vi "GitLog-to-CommitCluster.vi"(3 "Git Log In":string) -> (1 "Array":T1[](array[typedef]))   [LabVIEW 2013]
uses:
  CommitCluster.ctl
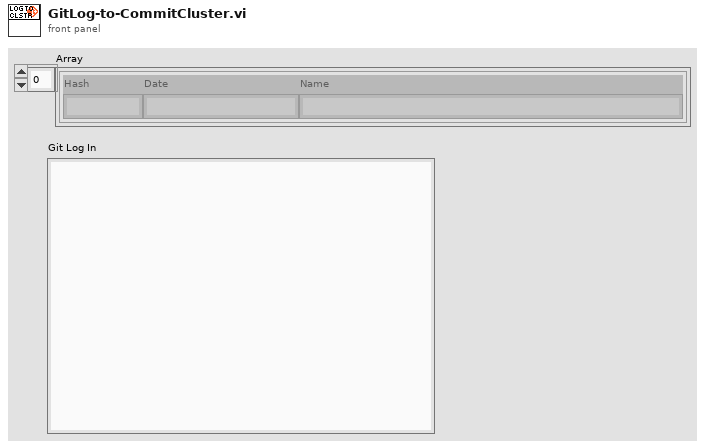
[diagram p1: front panel]
types:
  T1 = typedef "CommitCluster.ctl" = cluster{"Hash":string, "Date":string, "Name":string}
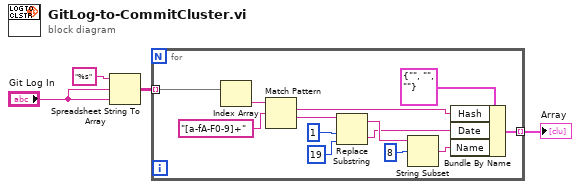
[diagram p0: block diagram]
diagram:
  n1 = Spreadsheet String To Array(format string="%s", spreadsheet string="Git Log In", array type (2D Dbl)="Git Log In") -> (array=w2:string[][])  [unwired: 1 in]
  n2 = for {
    tunnel: w2 -> [w11] mode=indexing
    tunnel: [w8] -> w1 mode=indexing
    n3 = Index Array(array=w11) -> (element=w10:string)  [unwired: 1 in]
    n4 = Match Pattern(string=w10, regular expression="[a-fA-F0-9]+") -> (match substring=w5:string, after substring=w14:string)  [unwired: 1 in, 2 out]
    n5 = Replace Substring(2:19 ("length (rest)"), 3:1 ("offset (0)"), 5:w14) -> (0:w7:string, 1:w12:string)  [unwired: 1 in]
    n6 = String Subset(string=w12, offset (0)=8) -> (substring=w6:string)  [unwired: 1 in]
    n7 = Bundle By Name(cluster=T1 {"Hash"="", "Date"="", "Name"=""} ("Commit"), "Hash"=w5, "Date"=w7, "Name"=w6) -> (w8:T1)
  }
  "Array" <- w1
